vi "Display.vi"(8 "error in (no error)":errorcluster, 10 "SubPnl Refnum":refnum<vi>, 11 "Slide in":refnum<class "Slide.lvclass">) -> (0 "error out":errorcluster, 3 "Slide out":refnum<class "Slide.lvclass">)   [LabVIEW 2017, in "Slide.lvclass"]
uses:
  Slide.lvclass
  Slide.lvclass/Slide.ctl
panel:
  out "2D Picture":picture
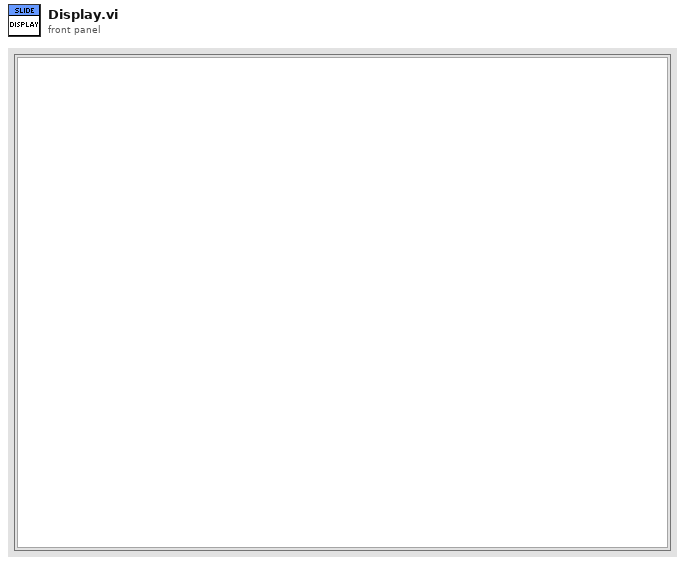
[diagram p1: front panel]
types:
  T1 = typedef "Slide.lvclass/SlideType.ctl" = enum16{"Image", "FP", "BD"}
  T2 = typedef "imagedata.ctl" = cluster{"image type":i32, "image depth":i32, "image":u8[], "mask":u8[], "colors":u32[], "Rectangle":cluster{"left":i16, "top":i16, "right":i16, "bottom":i16}}
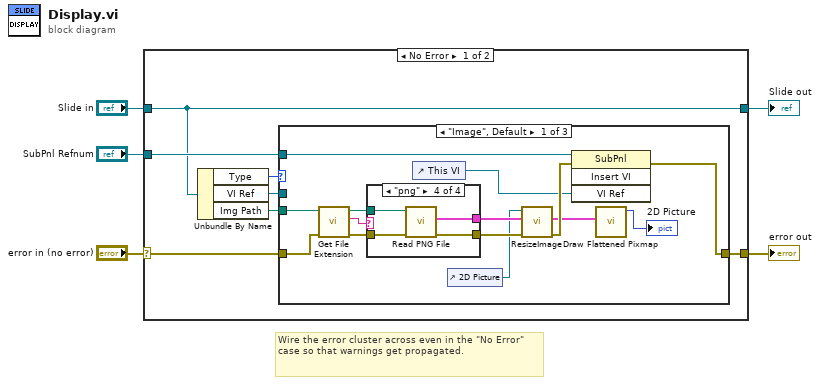
[diagram p0: block diagram]
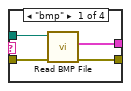
[diagram p2: hidden frame]
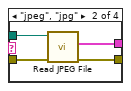
[diagram p3: hidden frame]
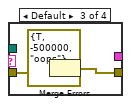
[diagram p4: hidden frame]
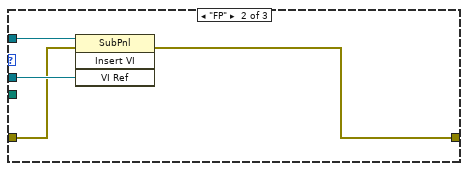
[diagram p5: hidden frame]
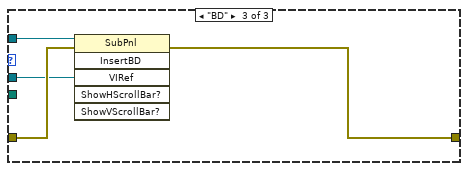
[diagram p6: hidden frame]
diagram:
  # "Wire the error cluster across even in the \"No Error\"\ncase so that warnings get propagated."
  n1 = case shown="No Error" "error in (no error)" {
    selector: "error in (no error)" -> [w12 w51]
    tunnel: [w7 w51] -> w4
    tunnel: [w10 w50] -> w2
    tunnel: "Slide in" -> [w10 w50]
    tunnel: "SubPnl Refnum" -> [w11 _]
    frame No Error {
      n2 = Unbundle By Name(w10) -> ("Type"=w9:T1, "VI Ref"=w8:refnum<vi>, "Img Path"=w6:path)
      n3 = case shown="\"Image\", Default" w9 {
        tunnel: w11 -> [w18 w45 w49]
        tunnel: w8 -> [_ w44 w46]
        tunnel: w12 -> [w24 w43 w48]
        tunnel: [w17 w42 w47] -> w7
        tunnel: w6 -> [w25 _ _]
        frame "Image", Default {
          n4 = call <vilib>:"Get File Extension.vi"("error in (no error)"=w24, "file"=w25) -> ("error out"=w19:errorcluster, "lowercase file extension"=w21:string, "dup file"=w20:path)  [unwired: 5 in, 2 out]
          n5 = case shown="\"png\"" w21 {
            tunnel: [w28 w31 _ w41] -> w23
            tunnel: w20 -> [w30 w33 _ w40]
            tunnel: w19 -> [w29 w34 w37 w39]
            tunnel: [w27 w32 w36 w38] -> w14
            frame "bmp" {
              n6 = call <vilib>:"Read BMP File.vi"("error in (no error)"=w29, "path to BMP file"=w30) -> ("error out"=w27:errorcluster, "image data"=w28:T2)  [unwired: 7 in, 1 out]
            }
            frame "jpeg", "jpg" {
              n7 = call <vilib>:"Read JPEG File.vi"("error in (no error)"=w34, "path to JPEG file"=w33) -> ("error out"=w32:errorcluster, "image data"=w31:T2)  [unwired: 7 in, 1 out]
            }
            frame Default {
              n8 = Merge Errors(errorcluster {"status"=TRUE, "code"=-500000, "source"="oops"} ("error constant"), w37) -> (w36:errorcluster)
            }
            frame "png" {
              n9 = call <vilib>:"Read PNG File.vi"("error in (no error)"=w39, "path to PNG file"=w40) -> ("error out"=w38:errorcluster, "image data"=w41:T2)  [unwired: 7 in, 1 out]
            }
          }
          n10 = control-ref of="This VI"() -> (w16:refnum<vi>)
          n11 = control-ref of="2D Picture"() -> (w13:refnum<vi>)
          n12 = call "ResizeImage.vi"("error in (no error)"=w14, "Image Data"=w23, "2D Picture Ref"=w13) -> ("error out"=w26:errorcluster, "Image Data (dup)"=w15:T2)  [unwired: 6 in, 1 out]
          n13 = invoke class="SubPnl" method="Insert VI"(reference=w18, error in=w26, "VI Ref"=w16) -> (error out=w17:errorcluster)  [unwired: 1 in, 3 out]
          n14 = call <vilib>:"Draw Flattened Pixmap.vi"("image data"=w15) -> ("new picture"=→"2D Picture":picture)  [unwired: 8 in]
        }
        frame "FP" {
          n15 = invoke class="SubPnl" method="Insert VI"(reference=w45, error in=w43, "VI Ref"=w44) -> (error out=w42:errorcluster)  [unwired: 1 in, 3 out]
        }
        frame "BD" {
          n16 = invoke class="SubPnl" method="InsertBD"(reference=w49, error in=w48, "VIRef"=w46) -> (error out=w47:errorcluster)  [unwired: 3 in, 5 out]
        }
      }
    }
    frame Error {
    }
  }
  "error out" <- w4
  "Slide out" <- w2
